vi "HapticSTM_Feedblackless_testdata.vi"() -> ()   [LabVIEW 2017]
uses:
  <vilib>/Analysis/3filter.llb/Filter Passband Type.ctl
  <vilib>/Utility/file.llb/Read Delimited Spreadsheet (DBL).vi
  <userlib>/HapticSTM/Feedbackless - Testdata/Project/feedbackless.lvproj/Proj/Feedbackless Folder/HapticSTM/GlobalClicksHeight.vi
  <userlib>/HapticSTM/Feedbackless - Testdata/Project/feedbackless.lvproj/Proj/Feedbackless Folder/HapticSTM/HapticSTM.lvlib
  <vilib>/ptbypt/NI_PtbyPt.lvlib
  <vilib>/Analysis/NI_AALBase.lvlib
panel:
  out "SeqString":string
  out "Seq":i32
  out "Raw and Scaled Z Positions":cluster{dbl, "Y":dbl}(graph)
  in  "Force Mode":u16(ring) items=["Stacked Logs", "Simple Log", "Linear"]
  out "Button":bool
  out "Filtered Current":dbl
  in  "Reset Clicks":bool
  out "Scaled Force and Current":cluster{dbl, "Filtered x":dbl, dbl}(graph)
  in  "Maximum (pA)":dbl=9000.0
  in  "Setpoint (pA)":dbl=100.0
  out "PLANE HEIGHT":dbl
  out "Current":dbl
  out "Origin Y":dbl
  out "Origin X":dbl
  out "Output Z":dbl
  out "Nano Z":dbl
  out "Width":dbl
  out "VY":dbl
  out "VZ":dbl
  out "VX":dbl
  in  "STOP":bool
  in  "START":bool
  out "Fy":dbl
  out "Fz":dbl
  out "phi":dbl
  out "psi":dbl
  out "Fx":dbl
  out "theta":dbl
  out "x":dbl
  out "y":dbl
  out "z":dbl
  in  "Fine adjust":dbl=3.5
  out "Clicks":i32
  out "Height":dbl
  # "Frame"
  # "Position"
  # "Sensitivity"
  # "Force"
  # "STM I/O"
  # "Angles"
  # "Current"
  # "Velocity"
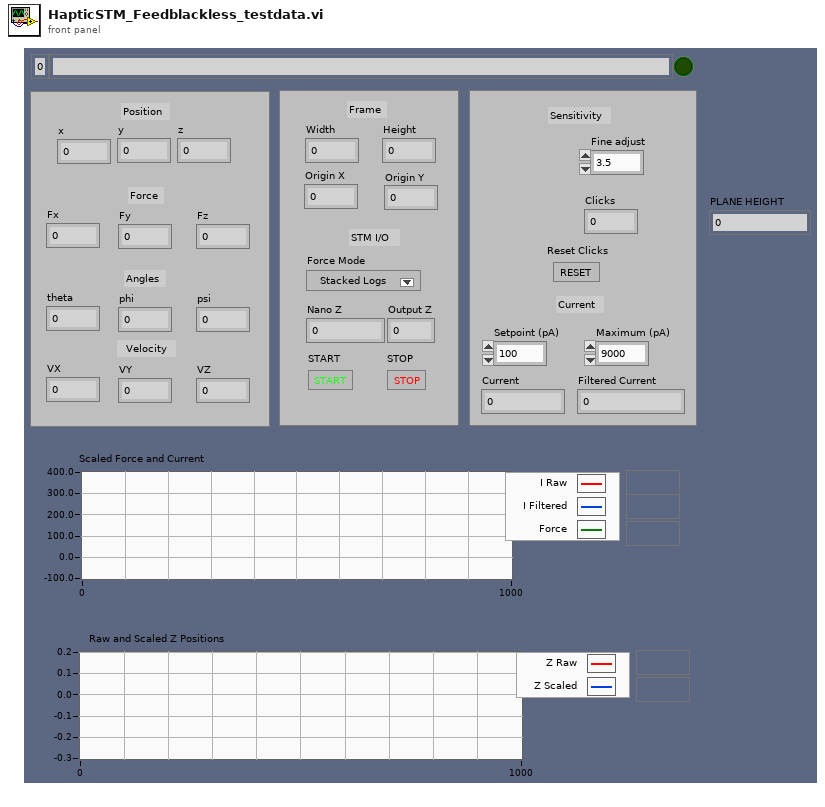
[diagram p1: front panel]
types:
  T1 = typedef "NI_AALBase.lvlib/Filter Passband Type.ctl" = enum32{"Lowpass", "Highpass", "Bandpass", "Bandstop"}
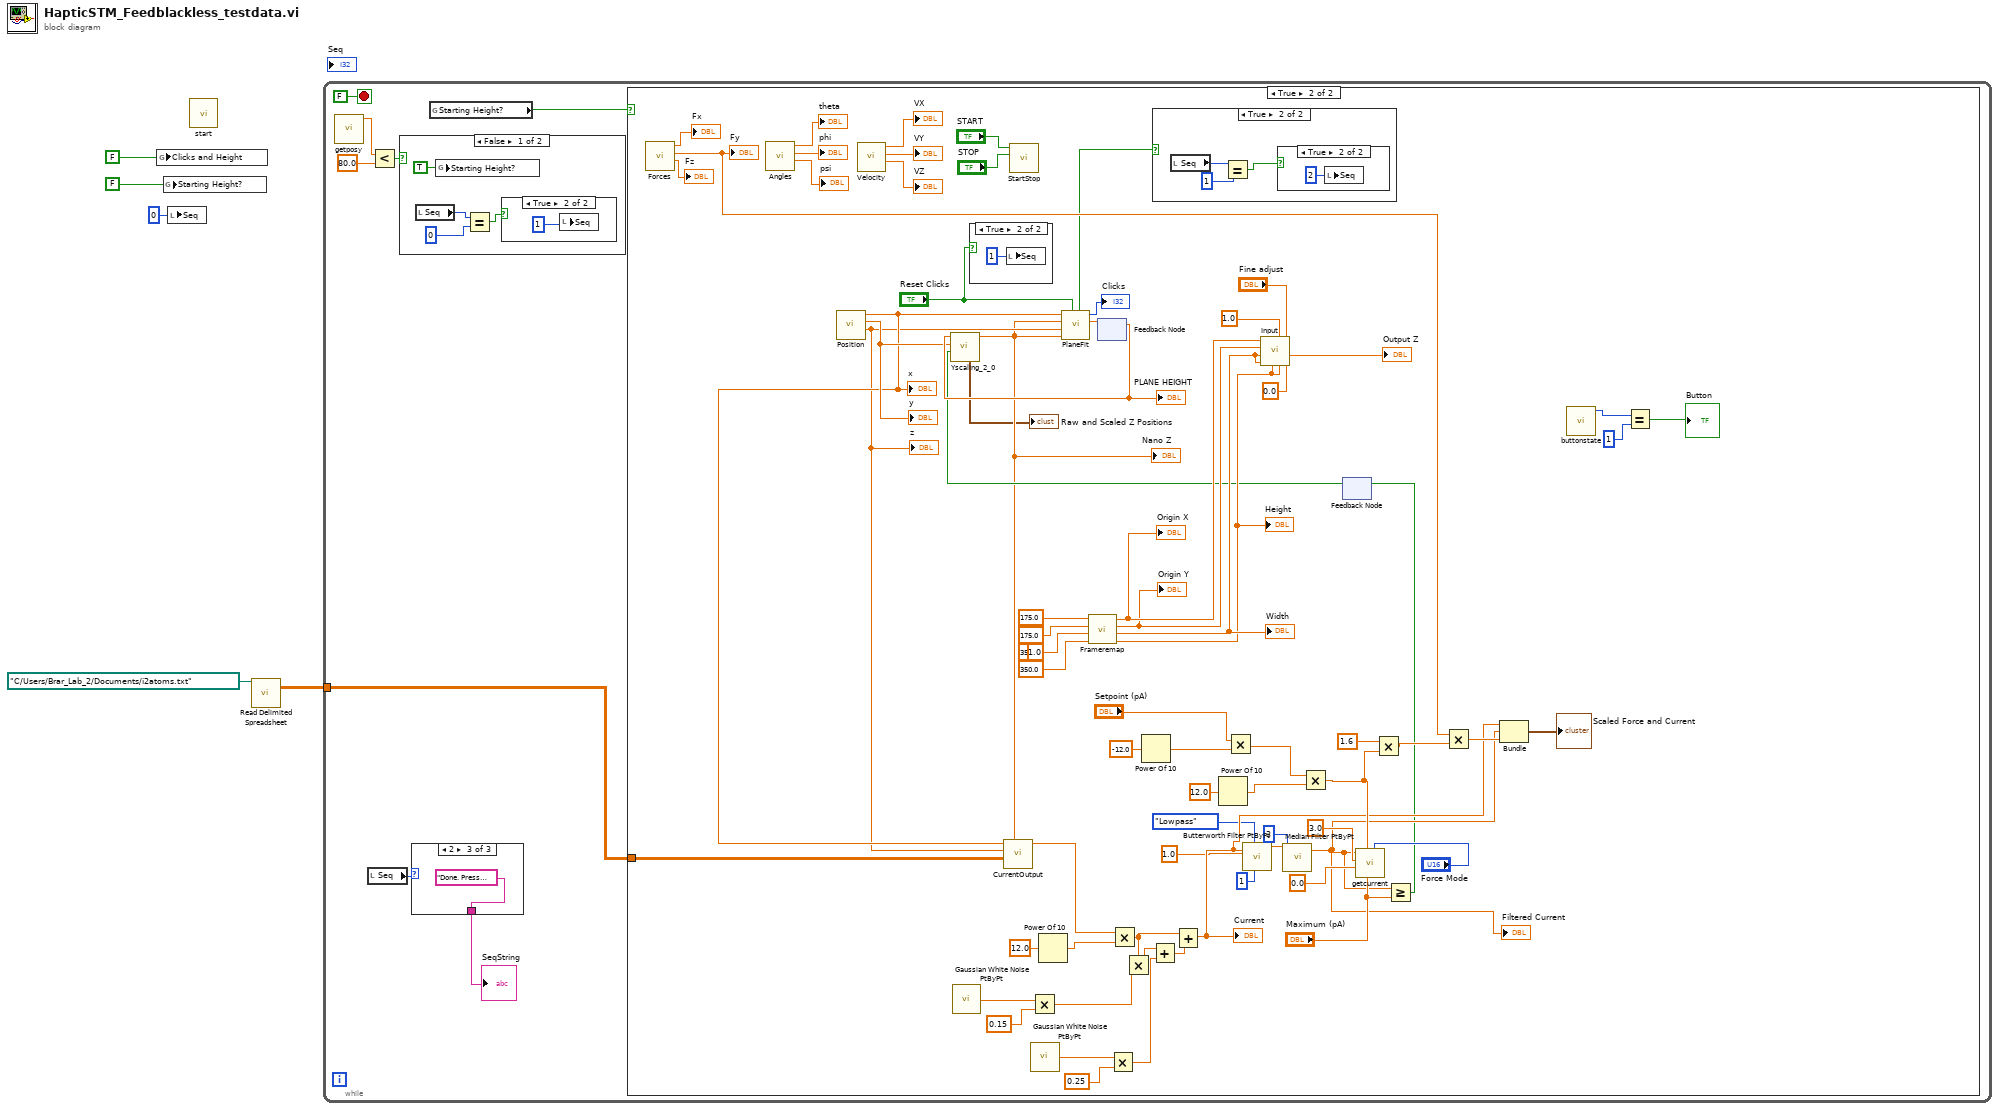
[diagram p0: block diagram]
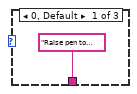
[diagram p2: hidden frame]
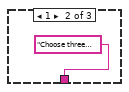
[diagram p3: hidden frame]
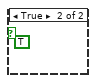
[diagram p5: hidden frame]
diagram:
  n1 = global write "GlobalClicksHeight.vi" "Clicks and Height"(FALSE ("Clicks and Height")) -> ()
  n2 = global write "GlobalClicksHeight.vi" "Starting Height?"(FALSE ("Clicks and Height")) -> ()
  n3 = local write "Seq"(0 ("Seq")) -> ()
  n4 = call <userlib>:"start.vi"() -> ()  [unwired: 11 in, 1 out]
  n5 = call-poly <vilib>:"Read Delimited Spreadsheet.vi"("file path (dialog if empty)"=path "C:/Users/Brar_Lab_2/Documents/i2atoms.txt") -> ("all rows"=w5:dbl[][])  [unwired: 9 in, 5 out]
  n6 = while {
    tunnel: w5 -> [w13]
    stop <- FALSE stop-if-true
    n7 = call <userlib>:"getposy.vi"() -> ("function return"=w12:dbl)  [unwired: 11 in]
    n8 = local read "Seq"() -> (w7:i32)
    n9 = Less?(x=w12, y=80.0) -> (x < y?=w10:bool)
    n10 = case shown="False" w10 {
      frame False {
        n11 = local read "Seq"() -> (w19:i32)
        n12 = global write "GlobalClicksHeight.vi" "Starting Height?"(TRUE ("Starting Height?")) -> ()
        n13 = Equal?(x=w19, y=0) -> (x = y?=w17:bool)
        n14 = case shown="True" w17 {
          frame False {
          }
          frame True {
            n15 = local write "Seq"(1 ("Seq")) -> ()
          }
        }
      }
      frame True {
        (unwired) TRUE ("Clicks and Height")
      }
    }
    n16 = case shown="2" w7 {
      tunnel: ["Raise pen to begin." "Choose three points, then raise the arm to plane." "Done. Press 'STOP' to stop at anytime."] -> w6
      frame 0, Default {
      }
      frame 1 {
      }
      frame 2 {
      }
    }
    "SeqString" <- w6
    n17 = global read "GlobalClicksHeight.vi" "Starting Height?"() -> (w9:bool)
    n18 = case shown="True" w9 {
      tunnel: w13 -> [_ w29]
      frame False {
      }
      frame True {
        (unwired) 1.0 ("FO X")
        n19 = call <userlib>:"Forces.vi"() -> ("Fz"=→"Fz":dbl, "Fy"=w58:dbl, "Fx"=→"Fx":dbl)  [unwired: 9 in]
        "Fy" <- w58
        n20 = call <userlib>:"Angles.vi"() -> ("psi"=→"psi":dbl, "phi"=→"phi":dbl, "theta"=→"theta":dbl)  [unwired: 9 in]
        n21 = call <userlib>:"Position.vi"() -> ("Z"=w30:dbl, "Y"=w44:dbl, "X"=w31:dbl)  [unwired: 9 in]
        "x" <- w31
        "y" <- w44
        "z" <- w30
        n22 = call <userlib>:"Velocity.vi"() -> ("VZ"=→"VZ":dbl, "VY"=→"VY":dbl, "VX"=→"VX":dbl)  [unwired: 9 in]
        n23 = call <vilib>:"Gaussian White Noise PtByPt.vi"() -> ("Gaussian white noise"=w57:dbl)  [unwired: 3 in]
        n24 = case shown="True" "Reset Clicks" {
          frame False {
          }
          frame True {
            n25 = local write "Seq"(1 ("Seq")) -> ()
          }
        }
        n26 = call <userlib>:"StartStop.vi"("STOP"="STOP", "START"="START") -> ()  [unwired: 10 in]
        n27 = Multiply(x=w57, y=0.15) -> (x*y=w55:dbl)
        n28 = call <vilib>:"Gaussian White Noise PtByPt.vi"() -> ("Gaussian white noise"=w52:dbl)  [unwired: 3 in]
        n29 = Power Of 10(x=12.0) -> (10^x=w76:dbl)
        n30 = call <userlib>:"Frameremap.vi"("FH"=350.0 ("FO X"), "FW"=350.0 ("FO X"), "FO Z"=175.0 ("FO X"), "FO X"=175.0) -> ("FH"=w82:dbl, "FW"=w83:dbl, "Z Origin"=w68:dbl, "X Origin"=w69:dbl)  [unwired: 4 in]
        "Height" <- w82
        "Width" <- w83
        "Origin X" <- w69
        "Origin Y" <- w68
        n31 = feedback #1() -> (w70:dbl)  [unwired: 1 in]
        "PLANE HEIGHT" <- w70
        n32 = Multiply(x=w52, y=0.25) -> (x*y=w48:dbl)
        n33 = Power Of 10(x=-12.0) -> (10^x=w65:dbl)
        n34 = Power Of 10(x=12.0) -> (10^x=w67:dbl)
        n35 = Multiply(x="Setpoint (pA)", y=w65) -> (x*y=w63:dbl)
        n36 = call <userlib>:"Input.vi"("Current * 10^input"=0.0, "Sensitivity"="Fine adjust", "Scopez"=w82, "Drag"=1.0, "FH"=w82, "FW"=w83, "Scopex"=w83, "Z origin"=w68, "X origin"=w69) -> ("Scaled Current"=→"Output Z":dbl)  [unwired: 2 in]
        n37 = Multiply(x=w63, y=w67) -> (x*y=w45:dbl)
        n38 = feedback #2() -> (w61:bool)  [unwired: 1 in]
        n39 = call <userlib>:"Yscaling_2_0.vi"("Current Maxed?"=w61, "Y"=w44, "Plane Height"=w70) -> ("y scaled"=w28:dbl, "Zpos Graph (nm)"=→"Raw and Scaled Z Positions":cluster{dbl, "function return":dbl})  [unwired: 7 in]
        "Nano Z" <- w28
        n40 = call <userlib>:"CurrentOutput.vi"("y scaled"=w28, "array"=w29, "Z Input"=w30, "X Input"=w31) -> ("Current Out"=w32:dbl)  [unwired: 7 in]
        n41 = call <userlib>:"PlaneFit.vi"("Reset Clicks"="Reset Clicks", "Y PEN"=w28, "Z"=w30, "Nano Z"=w28, "X"=w31) -> ("Plane Height (m)"=w79:dbl, "Clicks"=→"Clicks":i32, "Planing Done?"=w23:bool)  [unwired: 4 in]
        n42 = feedback-in #1(w79) -> ()
        n43 = Multiply(x=w32, y=w76) -> (x*y=w54:dbl)
        n44 = Multiply(x=w54, y=w55) -> (x*y=w49:dbl)
        n45 = Add(x=w49, y=w48) -> (x+y=w50:dbl)
        n46 = case shown="True" w23 {
          frame False {
          }
          frame True {
            n47 = local read "Seq"() -> (w98:i32)
            n48 = Equal?(x=w98, y=1) -> (x = y?=w96:bool)
            n49 = case shown="True" w96 {
              frame False {
              }
              frame True {
                n50 = local write "Seq"(2 ("Seq")) -> ()
              }
            }
          }
        }
        n51 = Add(x=w54, y=w50) -> (x+y=w40:dbl)
        "Current" <- w40
        n52 = call <vilib>:"Butterworth Filter PtByPt.vi"("order"=1, "filter type"=Filter_Passband_Type."Lowpass", "sampling freq: fs"=1.0, "x"=w40) -> ("Filtered x"=w36:dbl)  [unwired: 5 in, 1 out]
        n53 = call <vilib>:"Median Filter PtByPt.vi"("rank"=3, "x"=w36) -> ("Filtered x"=w35:dbl)  [unwired: 2 in, 1 out]
        "Filtered Current" <- w35
        n54 = call <userlib>:"getcurrent.vi"("forcemode"="Force Mode", "maxcurrentin"="Maximum (pA)", "setpoint"=w45, "minforcey"=0.0, "maxforcey"=3.0, "currentin"=w35) -> ()  [unwired: 6 in]
        n55 = Multiply(x=1.6 ("y"), y=w45) -> (x*y=w46:dbl)
        n56 = Greater Or Equal?(x=w35, y="Maximum (pA)") -> (x >= y?=w27:bool)
        n57 = feedback-in #2(w27) -> ()
        n58 = Multiply(x=w58, y=w46) -> (x*y=w53:dbl)
        n59 = Bundle(w40, "Filtered x"=w35, w53) -> (→"Scaled Force and Current":cluster{dbl, "Filtered x":dbl, dbl})  [unwired: 1 in]
        n60 = call <userlib>:"buttonstate.vi"() -> ("function return"=w43:i32)  [unwired: 11 in]
        n61 = Equal?(x=w43, y=1) -> (x = y?=→"Button":bool)
      }
    }
  }
